vi "Update Channels.vi"(8 "error in":errorcluster, 10 "Channels to Create":T2[](array[typedef]), 11 "VI Map":T1) -> (0 "error out":errorcluster)   [LabVIEW 2021, in "Plugin Generator.lvlib"]
uses:
  Plugin Generator.lvlib
  <vilib>/CIF Foundation/CIF Core/Channels/ChannelRegistrar/typedef/Channel Definition for Scripting.ctl
  <vilib>/CIF Foundation/CIF Channels Core/CIFChannels/Typedef/Direction.ctl
  <vilib>/CIF Foundation/CIF Core/Channels/ChannelRegistrar/typedef/Registered Channel Types.ctl
  <vilib>/CIF Foundation/CIF LabVIEW Scripting/LV Scripting/Typedef/VI Map.ctl
  <vilib>/CIF Foundation/CIF Core/Channels/ChannelRegistrar/typedef/Channel Definition.ctl
  <vilib>/Utility/traverseref.llb/TRef TravTarget.ctl
  <vilib>/CIF Foundation/CIF LabVIEW Scripting/LV Scripting/Typedef/Errors.ctl
  <vilib>/CIF Foundation/CIF Utilities/Errors/Append Error Location.vi
  <vilib>/Utility/traverseref.llb/VI Scripting - Traverse.lvlib
  <vilib>/CIF Foundation/CIF Core/Channels/ChannelRegistrar/ChannelRegistrar.lvlib
  <vilib>/CIF Foundation/CIF Channels Core/CIFChannels/CIFChannels.lvclass
  <vilib>/CIF Foundation/CIF LabVIEW Scripting/Update Enum/Update Enum.lvlib
  <vilib>/CIF Foundation/CIF LabVIEW Scripting/LV Scripting/LV Scripting Utilities.lvlib
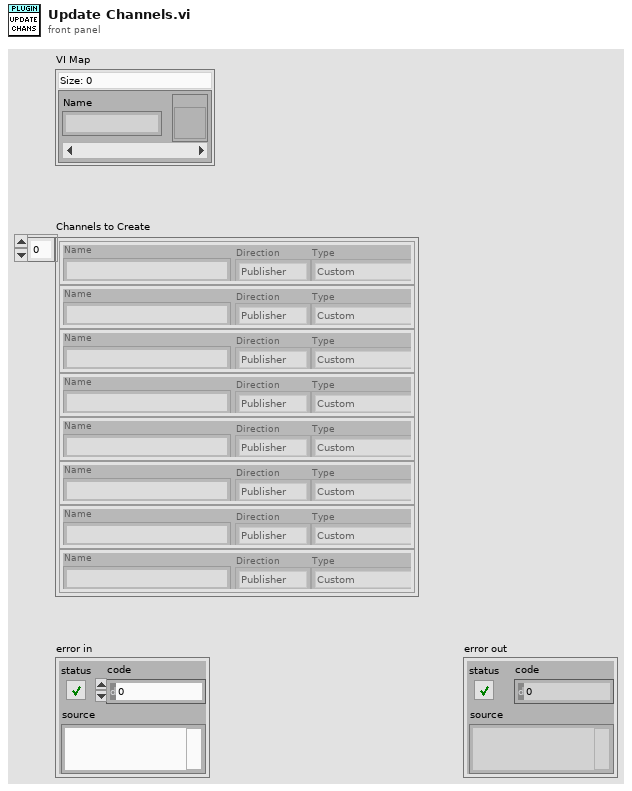
[diagram p1: front panel]
types:
  T1 = typedef "LV Scripting Utilities.lvlib/VI Map.ctl" = map{string, refnum<vi>}
  T2 = typedef "ChannelRegistrar.lvlib/Channel Definition for Scripting.ctl" = cluster{"Name":string, "Direction":T3, "Type":T4}
  T3 = typedef "CIFChannels.lvclass/Direction.ctl" = enum16{"Publisher", "Subscriber"}
  T4 = typedef "ChannelRegistrar.lvlib/Registered Channel Types.ctl" = enum16{"Custom", "Double_Tag", "I64_Tag", "U64_Tag", "U8_FIFO", "CAN_FIFO", "L2Enet_FIFO", "DAQ_FIFO", "Universal_FIFO", "String_Tag"}
  T5 = typedef "ChannelRegistrar.lvlib/Channel Definition.ctl" = cluster{"Name":string, "Direction":T3, "Type":T4, "Custom Config Data":u8[]}
  T6 = typedef "TRef TravTarget.ctl" = enum16{"FP", "BD", "Other"}
  T7 = typedef "Errors.ctl" = enum16{"Missing Version Changes", "Item not found"}
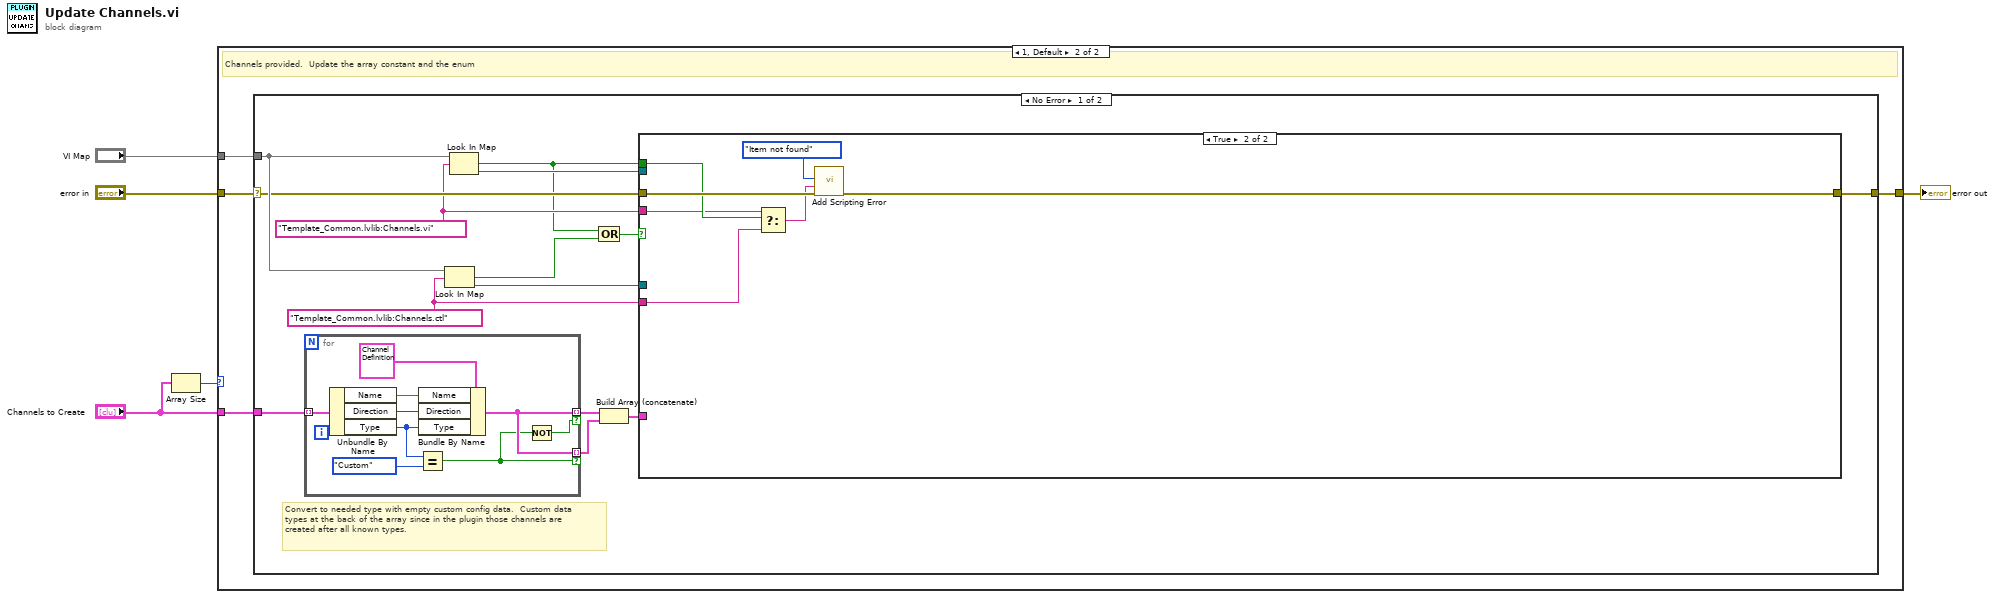
[diagram p0: block diagram]
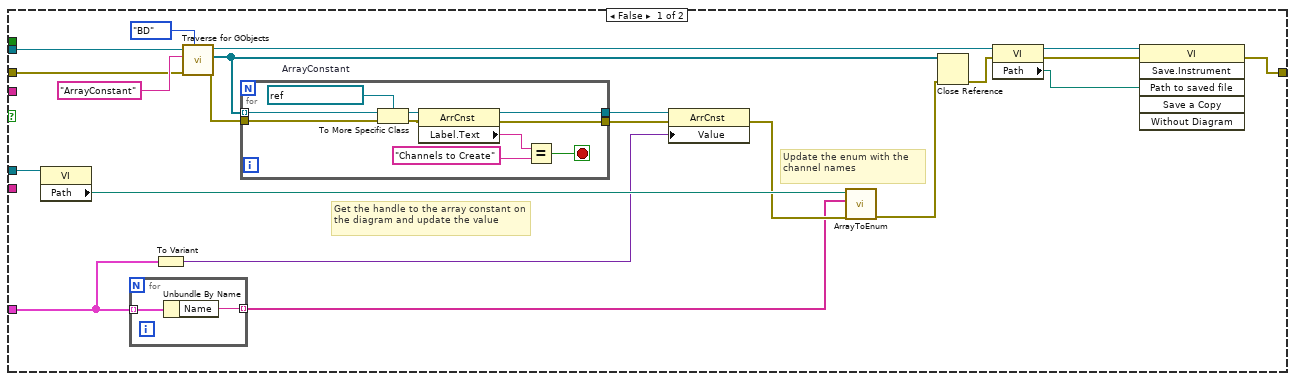
[diagram p3: hidden frame]
diagram:
  n1 = Array Size(array="Channels to Create") -> (size(s)=w1:i32)
  n2 = case shown="1, Default" w1 {
    tunnel: "VI Map" -> [_ w10]
    tunnel: "error in" -> [w6 w9]
    tunnel: [w6 w8] -> w3
    tunnel: "Channels to Create" -> [_ w7]
    frame 0 {
      # "No channel list provided. Skip scripting"
    }
    frame 1, Default {
      # "Channels provided.  Update the array constant and the enum"
      n3 = case shown="No Error" w9 {
        selector: w9 -> [w17 w74]
        tunnel: [w24 w74] -> w8
        tunnel: w10 -> [w22 _]
        tunnel: w7 -> [w18 _]
        frame No Error {
          w15 = "Template_Common.lvlib:Channels.ctl" ("String")
          w16 = "Template_Common.lvlib:Channels.vi" ("String")
          # "Convert to needed type with empty custom config data.  Custom data types at the back of the array since in the plugin those channels are created after all known types."
          n4 = for {
            tunnel: w18 -> [w33] mode=indexing
            tunnel: [w27] -> w13 mode=indexing if=w25
            tunnel: [w27] -> w12 mode=indexing if=w26
            n5 = Unbundle By Name(w33) -> ("Name"=w31:string, "Direction"=w30:T3, "Type"=w29:T4)
            n6 = Equal?(x=w29, y=Registered_Channel_Types."Custom") -> (x = y?=w26:bool)
            n7 = Bundle By Name(cluster=T5 {"Name"="testme", "Direction"=enum."Subscriber", "Type"=enum."L2Enet_FIFO", "Custom Config Data"=[]} ("Channel Definition"), "Name"=w31, "Direction"=w30, "Type"=w29) -> (w27:T5)
            n8 = Not(x=w26) -> (.not. x?=w25:bool)
          }
          n9 = Look In Map(map=w22, key=w15) -> (key not found?=w21:bool, value=w19:refnum<vi>)  [unwired: 1 in]
          n10 = Look In Map(map=w22, key=w16) -> (key not found?=w14:bool, value=w23:refnum<vi>)  [unwired: 1 in]
          n11 = Compound Arithmetic op=OR(w14, w21) -> (w20:bool)
          n12 = Build Array (concatenate)(w13, w12) -> (w11:T5[])
          n13 = case shown="True" w20 {
            tunnel: [w46 w71] -> w24
            tunnel: w23 -> [w45 _]
            tunnel: w17 -> [w44 w72]
            tunnel: w19 -> [w40 _]
            tunnel: w11 -> [w35 _]
            tunnel: w16 -> [_ w69]
            tunnel: w15 -> [_ w68]
            tunnel: w14 -> [_ w70]
            frame False {
              # "Update the enum with the channel names"
              # "Get the handle to the array constant on the diagram and update the value"
              n14 = property class="VI"(reference=w40) -> ("Path"=w39:path)  [unwired: 1 in, 2 out]
              n15 = for {
                tunnel: w35 -> [w56] mode=indexing
                tunnel: [w55] -> w34 mode=indexing
                n16 = Unbundle By Name(w56) -> ("Name"=w55:string)
              }
              n17 = To Variant(anything=w35) -> (Variant=w36:variant)
              n18 = call <vilib>:"Traverse for GObjects.vi"("Traverse Target"=TRef_TravTarget."BD", "error in (no error)"=w44, "Class Name"="ArrayConstant", "VI Refnum"=w45) -> ("error out"=w43:errorcluster, "References"=w52:refnum<vi>[], "dup VI Refnum"=w49:refnum<vi>)  [unwired: 4 in, 1 out]
              n19 = for {
                tunnel: w52 -> [w66] mode=indexing
                tunnel: [w63] -> w42
                tunnel: [w62] -> w41
                tunnel: w43 -> [w61]
                stop <- w57 stop-if-true
                w65 = refnum<vi> refnum  # ArrayConstant
                n20 = To More Specific Class(target class=w65, reference=w66, error in=w61) -> (specific class reference=w64:refnum<vi>, error out=w60:errorcluster)
                n21 = property class="ArrCnst"(reference=w64, error in=w60) -> (reference out=w63:refnum<vi>, error out=w62:errorcluster, "Label.Text"=w59:string)
                n22 = Equal?(x=w59, y="Channels to Create") -> (x = y?=w57:bool)
              }
              n23 = property class="ArrCnst"(reference=w42, error in=w41, "Value"=w36) -> (error out=w38:errorcluster)  [unwired: 1 out]
              n24 = call <vilib>:"ArrayToEnum.vi"("Error In"=w38, "Enum Strings"=w34, "Enum Path"=w39) -> ("Error Out"=w37:errorcluster)  [unwired: 8 in]
              n25 = Close Reference(reference=w52, error in (no error)=w37) -> (error out=w48:errorcluster)
              n26 = property class="VI"(reference=w49, error in=w48) -> (reference out=w54:refnum<vi>, error out=w53:errorcluster, "Path"=w47:path)
              n27 = invoke class="VI" method="Save.Instrument"(reference=w54, error in=w53, "Path to saved file"=w47) -> (error out=w46:errorcluster)  [unwired: 3 in, 5 out]
            }
            frame True {
              n28 = Select(t=w69, s=w70, f=w68) -> (s? t:f=w67:string)
              n29 = call <vilib>:"Add Scripting Error.vi"("error in (no error)"=w72, "String to Append"=w67, "Error"=Errors."Item not found") -> ("error out"=w71:errorcluster)  [unwired: 8 in]
            }
          }
        }
        frame Error {
        }
      }
    }
  }
  "error out" <- w3
